vi "oa_Convert Resampled Signal to Waveform Signal.vi"(0 "resampled signal":cluster{"r0":dbl, "dr":dbl, "Y":dbl[]}={"r0"=0.0, "dr"=1.0, "Y"=[]} {"r0" format="%.2p"; "dr" format="%.2p"; "Y" format="%.2f"}, 11 "error in":errorcluster) -> (4 "signal in":waveform(dbl), 15 "error out":errorcluster)   [LabVIEW 2017, in "SoundVib_RefDataProcess.lvlib"]
uses:
  <vilib>/addons/Sound and Vibration/Order Analysis/Referece Data Processing/SoundVib_RefDataProcess.lvlib
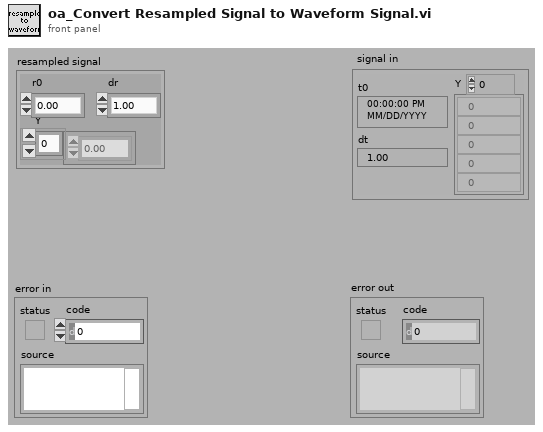
[diagram p1: front panel]
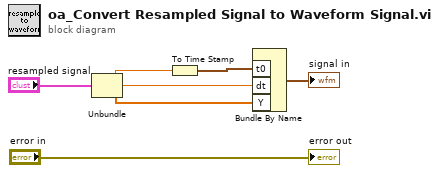
[diagram p0: block diagram]
diagram:
  n1 = Unbundle("resampled signal") -> ("r0"=w3:dbl, "dr"=w4:dbl, "Y"=w5:dbl[])
  n2 = To Time Stamp(1:w3) -> (0:w2:timestamp)
  n3 = Bundle By Name("t0"=w2, "dt"=w4, "Y"=w5) -> (→"signal in":waveform(dbl))  [unwired: 1 in]
  "error out" <- "error in"
